vi "응답 프레임.vi"(11 "응답":string) -> (1 "에러 코드":string, 2 "U16 배열":u16[](array[numeric])=[4660, 22136] format="%.0x", 3 "데이터 개수":string="04")   [LabVIEW 2014]
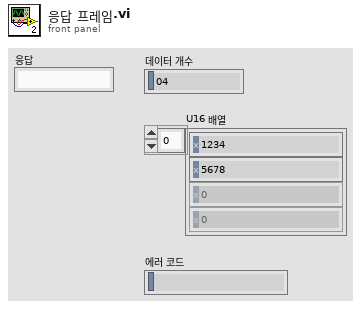
[diagram p1: front panel]
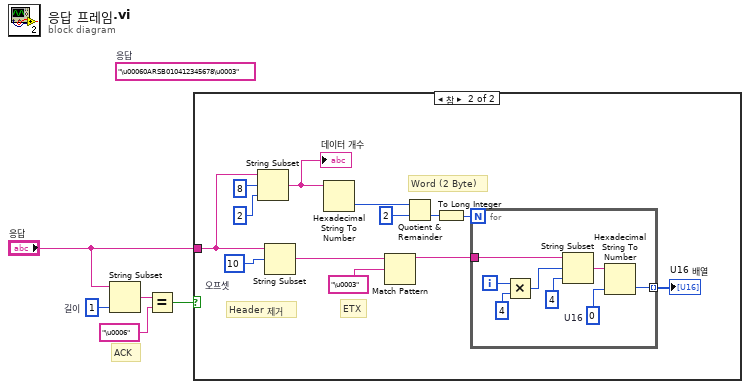
[diagram p0: block diagram]
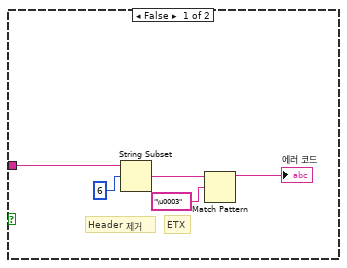
[diagram p2: hidden frame]
diagram:
  (unwired) "\u00060ARSB010412345678\u0003"  # 응답
  w2 = 1  # 길이
  # "ACK"
  n1 = String Subset(string="응답", length (rest)=w2) -> (substring=w3:string)  [unwired: 1 in]
  n2 = Equal?(x=w3, y="\u0006") -> (x = y?=w5:bool)
  n3 = case shown="참" w5 {
    tunnel: "응답" -> [w10 w18]
    frame False {
      # "Header 제거"
      # "ETX"
      n4 = String Subset(string=w10, offset (0)=6 ("오프셋(0)")) -> (substring=w8:string)  [unwired: 1 in]
      n5 = Match Pattern(string=w8, regular expression="\u0003" ("정규식")) -> (before substring=→"에러 코드":string)  [unwired: 1 in, 3 out]
    }
    frame True {
      w23 = 10  # 오프셋
      # "Word (2 Byte)"
      # "Header 제거"
      # "ETX"
      n6 = String Subset(string=w18, offset (0)=8, length (rest)=2 ("길이(나머지)")) -> (substring=w20:string)
      "데이터 개수" <- w20
      n7 = String Subset(string=w18, offset (0)=w23) -> (substring=w17:string)  [unwired: 1 in]
      n8 = Hexadecimal String To Number(string=w20) -> (number=w14:u32)  [unwired: 2 in, 1 out]
      n9 = Match Pattern(string=w17, regular expression="\u0003") -> (before substring=w15:string)  [unwired: 1 in, 3 out]
      n10 = Quotient & Remainder(x=w14, y=u32 2) -> (floor(x/y)=w12:u32)  [unwired: 1 out]
      n11 = To Long Integer(number=w12) -> (32bit integer=w11:i32)
      n12 = for {
        N: w11 -> [_]
        tunnel: w15 -> [w31]
        tunnel: [w26] -> w19 mode=indexing
        i -> [w30]
        w24 = u16 0  # U16
        n13 = Multiply(x=w30, y=4) -> (x*y=w29:i32)
        n14 = String Subset(string=w31, offset (0)=w29, length (rest)=4 ("y")) -> (substring=w27:string)
        n15 = Hexadecimal String To Number ("16진수 문자열을 숫자로")(string=w27, default (0uL)=w24) -> (number=w26:u16)  [unwired: 1 in, 1 out]
      }
      "U16 배열" <- w19
    }
  }
